vi "Get Collision Type.vi"(7 "Combination in":string[](array[string]), 9 "GB Components in":refnum<class "Game Board Component.lvclass">[](array[class]), 11 "Movable in":refnum<class "Movable.lvclass">) -> (2 "Collision out":refnum<class "Collision.lvclass">, 5 "Combination out":string[](array[string]))   [LabVIEW 2021, in "Movable.lvclass"]
doc: "MIT Licence\nCopyright (c) 2024 David Grollier"
uses:
  Movable.lvclass
  Collision/Collision.lvclass
  Game Board Component.lvclass
  Collision/Ball-Edge/Ball-Edge.lvclass
  C:/Users/David/Documents/GameSoccerSpace/Source/Collision/Collision.lvclass
  Collision/Ball-Ball/Ball-Ball.lvclass
  Collision/Ball-Goal Post/Ball-Goal Post.lvclass
  <vilib>/Utility/error.llb/Error Cluster From Error Code.vi
  <vilib>/ErrorRing/Error Ring.xnode
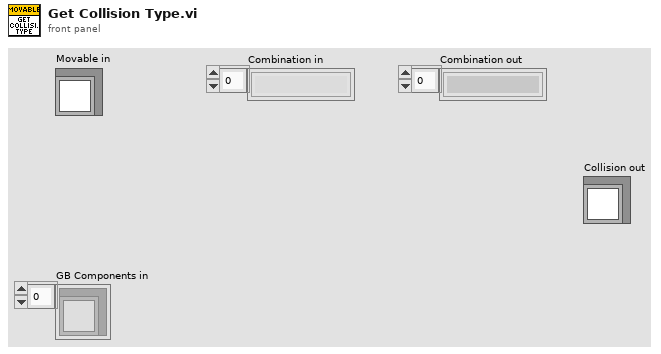
[diagram p1: front panel]
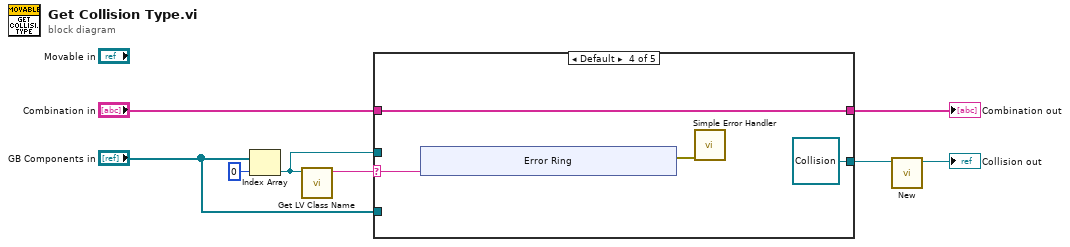
[diagram p0: block diagram]
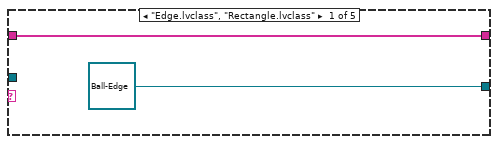
[diagram p2: hidden frame]
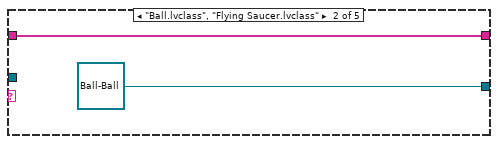
[diagram p3: hidden frame]
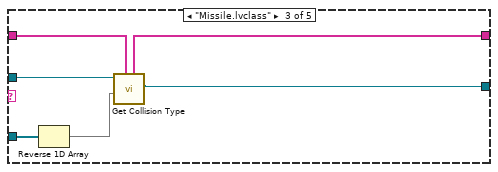
[diagram p4: hidden frame]
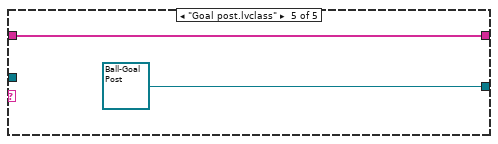
[diagram p5: hidden frame]
diagram:
  n1 = Index Array(array="GB Components in", index=0) -> (element=w4:refnum<class "Game Board Component.lvclass">)
  n2 = call <vilib>:"Get LV Class Name.vi"("object"=w4) -> ("class name"=w7:string)  [unwired: 9 in, 1 out]
  n3 = case shown="Default" w7 {
    selector: w7 -> [_ _ _ w20 _]
    tunnel: "Combination in" -> [w10 w12 w16 w22 w31]
    tunnel: [w10 w12 w15 w22 w31] -> w5
    tunnel: w4 -> [_ _ w18 _ _]
    tunnel: "GB Components in" -> [_ _ w17 _ _]
    tunnel: [refnum<class "Ball-Edge.lvclass"> refnum ("Ball-Edge.lvclass") refnum<class "Ball-Ball.lvclass"> refnum ("Ball-Ball.lvclass") w14 refnum<class "Collision.lvclass"> refnum ("Collision in") refnum<class "Ball-Goal Post.lvclass"> refnum ("Ball-Goal Post.lvclass")] -> w2
    frame "Edge.lvclass", "Rectangle.lvclass" {
    }
    frame "Ball.lvclass", "Flying Saucer.lvclass" {
    }
    frame "Missile.lvclass" {
      n4 = Reverse 1D Array(array=w17) -> (reversed array=w13:refnum<class "Game Board Component.lvclass">[])
      n5 = call-dynamic "Get Collision Type.vi"("Combination in"=w16, "GB Components in"=w13, "Game Board Component in"=w18) -> ("Collision out"=w14:refnum<class "Collision.lvclass">, "Combination out"=w15:string[])  [unwired: 7 in]
    }
    frame Default {
      n6 = xnode "Error Ring"("parameter 0"=w20) -> ("error out"=w19:errorcluster)
      n7 = call <vilib>:"Simple Error Handler.vi"("error in (no error)"=w19) -> ()  [unwired: 4 in, 5 out]
    }
    frame "Goal post.lvclass" {
    }
  }
  "Combination out" <- w5
  n8 = call "New.vi"("Collision in"=w2) -> ("Collision out"=→"Collision out":refnum<class "Collision.lvclass">)  [unwired: 10 in]
